vi "Startup 1.vi"(6 "LabVIEW Web Service":refnum<class "Web Service.lvclass">) -> ()   [LabVIEW 2015]
uses:
  <vilib>/wsapi/Web Service.lvclass
  Source/Classes/Request/Request.lvclass/Request.ctl
  Source/Classes/Request/Read method.vi
  Source/Classes/Request/Read params.vi
  <vilib>/National Instruments/JSON Support for LabVIEW/JSON Data Classes/JSON String/New JSON String.vi
  Source/Classes/Server/Add Response (Method Not Found from Request).vi
  Source/Classes/Server/Add Response (Result from Request).vi
  Source/Classes/Server/Add Response (Invalid Params from Request).vi
  <vilib>/National Instruments/JSON Support for LabVIEW/JSON Data Classes/JSON Datatype/To More Specific Type (Array).vi
  <vilib>/National Instruments/JSON Support for LabVIEW/JSON Data Classes/JSON Array/Index Array (Numeric).vi
  <vilib>/National Instruments/JSON Support for LabVIEW/JSON Data Classes/JSON Numeric/Read value (Numeric).vi
  <vilib>/National Instruments/JSON Support for LabVIEW/JSON Data Classes/JSON Numeric/New JSON Numeric.vi
  Source/Classes/Server/Add Response (Server Error from Request).vi
  <vilib>/National Instruments/JSON Support for LabVIEW/JSON Data Classes/JSON Datatype/JSON Datatype.lvclass
  Source/Classes/params/params.lvclass
  Source/Classes/Server/JSONRPC Server.lvclass
  Source/Classes/Request/Request.lvclass
  <vilib>/National Instruments/JSON Support for LabVIEW/JSON Data Classes/JSON Basic Type/JSON Basic Type.lvclass
  <vilib>/National Instruments/JSON Support for LabVIEW/JSON Data Classes/JSON Numeric/JSON Numeric.lvclass
  <vilib>/National Instruments/JSON Support for LabVIEW/JSON Data Classes/JSON String/JSON String.lvclass
  <vilib>/National Instruments/JSON Support for LabVIEW/JSON Data Classes/JSON Array/JSON Array.lvclass
panel:
  out "String":string
  in  "error in (no error)":errorcluster
  out "error out":errorcluster
  # "Use the web service input terminal to call the VIs on the Service subpalette of the Web Services palette. Do not remove it from the connector pane unless you don't need access to the palette."
  # "Any additional terminals added to the connector pane of a startup VI will be ignored."
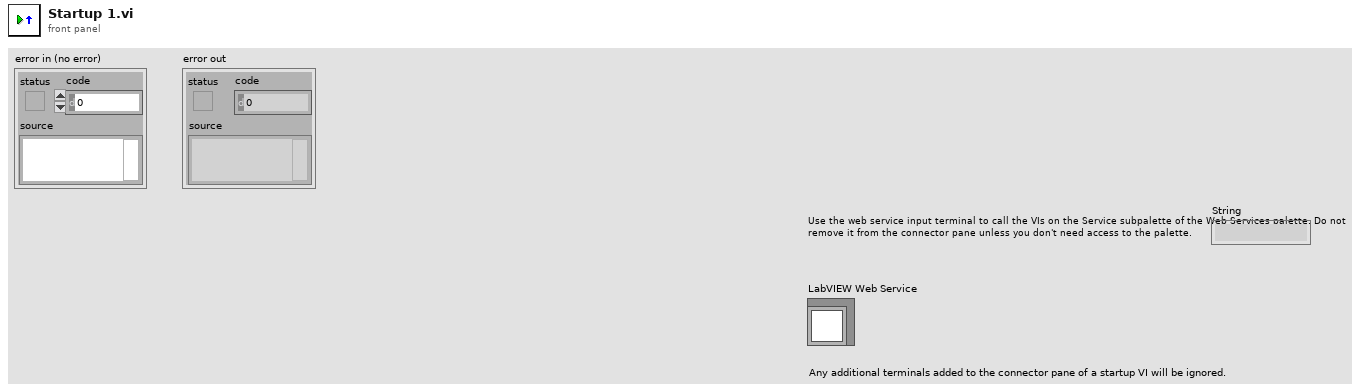
[diagram p1: front panel]
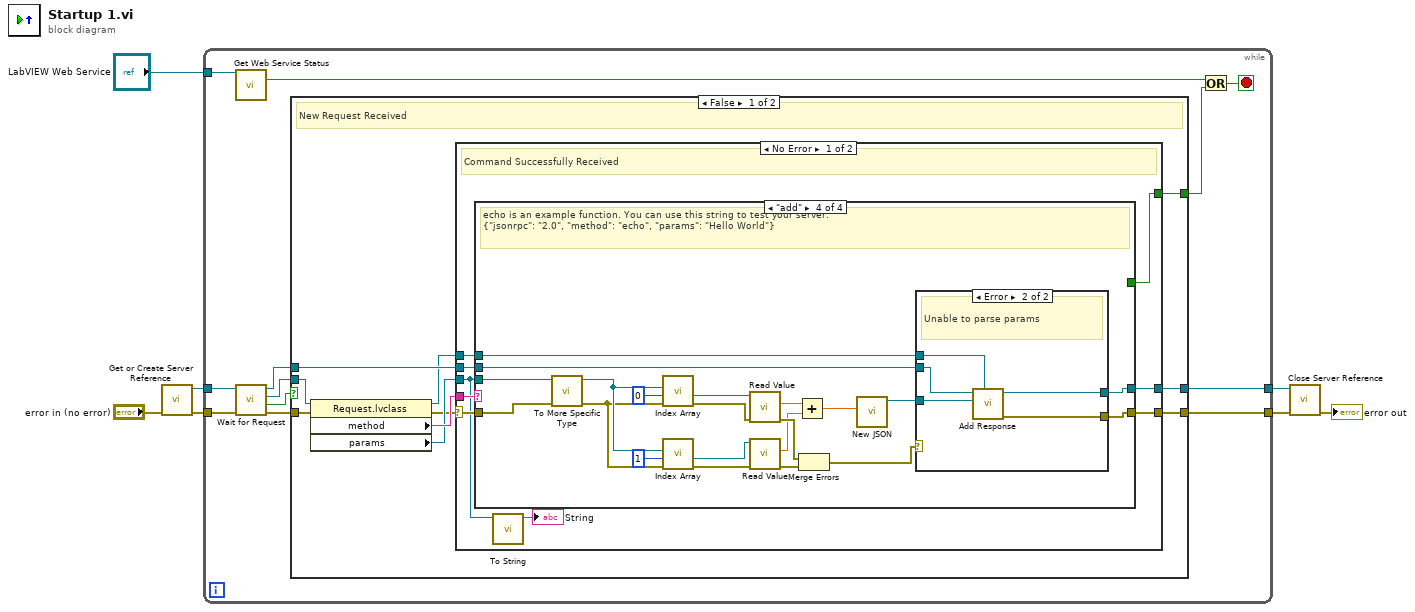
[diagram p0: block diagram]
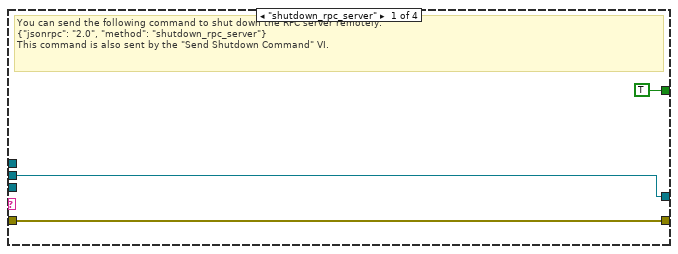
[diagram p2: hidden frame]
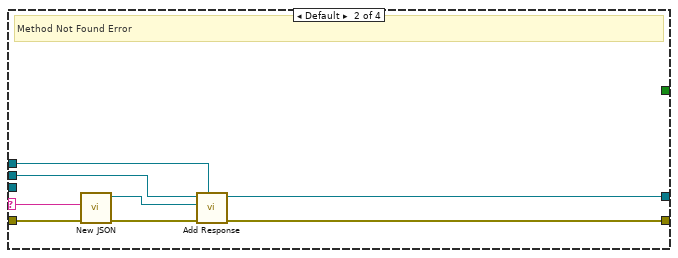
[diagram p3: hidden frame]
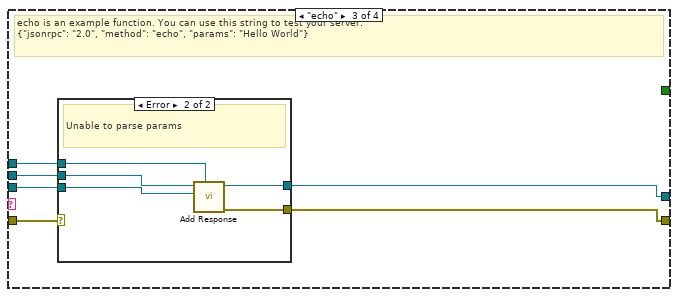
[diagram p4: hidden frame]
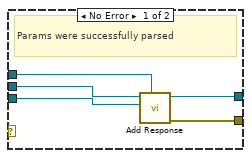
[diagram p5: hidden frame]
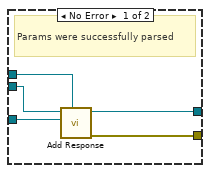
[diagram p6: hidden frame]
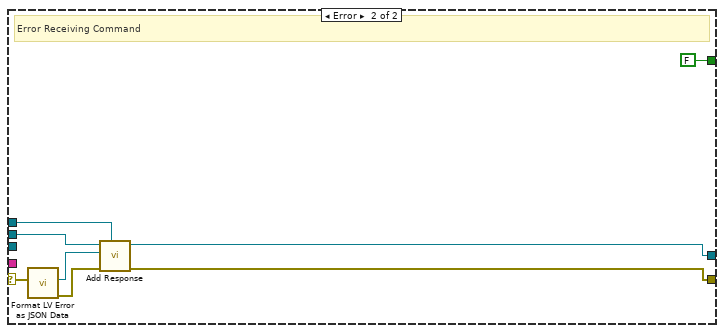
[diagram p7: hidden frame]
diagram:
  n1 = call "Get or Create Server Reference.vi"("error in (no error)"="error in (no error)") -> ("error out"=w6:errorcluster, "Server Out"=w7:refnum<class "JSONRPC Server.lvclass">)  [unwired: 9 in]
  n2 = while {
    tunnel: w7 -> [w19]
    tunnel: w6 -> [w15]
    tunnel: [w11] -> w4
    tunnel: [w13] -> w5
    tunnel: "LabVIEW Web Service" -> [w8]
    stop <- w10 stop-if-true
    n3 = call <vilib>:"Get Web Service Status.vi"("LabVIEW Web Service"=w8) -> ("service stopping?"=w9:bool)  [unwired: 12 in, 2 out]
    n4 = call "Wait for Request.vi"("error in (no error)"=w15, "Server in"=w19) -> ("error out"=w14:errorcluster, "timed out?"=w16:bool, "Request"=w17:refnum<class "Request.lvclass">, "Server out"=w18:refnum<class "JSONRPC Server.lvclass">)  [unwired: 6 in]
    n5 = case shown="False" w16 {
      tunnel: w18 -> [w22 w105]
      tunnel: w17 -> [w29 _]
      tunnel: w14 -> [w26 w106]
      tunnel: [w24 w106] -> w11
      tunnel: [w23 _] -> w12
      tunnel: [w21 w105] -> w13
      frame False {
        # "New Request Received"
        n6 = property class="Request.lvclass"(reference=w29, error in=w26) -> (reference out=w20:refnum<class "Request.lvclass">, error out=w25:errorcluster, "method"=w28:string, "params"=w27:refnum<class "JSON Datatype.lvclass">)
        n7 = case shown="No Error" w25 {
          selector: w25 -> [w37 w98]
          tunnel: w28 -> [w38 _]
          tunnel: w27 -> [w31 _]
          tunnel: [w36 w101] -> w24
          tunnel: [w35 FALSE] -> w23
          tunnel: w22 -> [w34 w103]
          tunnel: [w33 w102] -> w21
          tunnel: w20 -> [w32 w104]
          frame No Error {
            # "Command Successfully Received"
            n8 = case shown="\"add\"" w38 {
              selector: w38 -> [_ w45 _ _]
              tunnel: w31 -> [_ _ w51 w82]
              tunnel: w37 -> [w40 w44 w50 w80]
              tunnel: [w40 w47 w53 w84] -> w36
              tunnel: [TRUE _ _ _] -> w35
              tunnel: w34 -> [w39 w49 w55 w86]
              tunnel: [w39 w46 w54 w85] -> w33
              tunnel: w32 -> [_ w48 w52 w83]
              frame "shutdown_rpc_server" {
                # "You can send the following command to shut down the RPC server remotely:\n{\"jsonrpc\": \"2.0\", \"method\": \"shutdown_rpc_server\"}\nThis command is also sent by the \"Send Shutdown Command\" VI."
              }
              frame Default {
                # "Method Not Found Error"
                n9 = call-poly <vilib>:"New JSON.vi"("error in (no error)"=w44, "value"=w45) -> ("error out"=w43:errorcluster, "JSON String out"=w42:refnum<class "JSON String.lvclass">)  [unwired: 8 in]
                n10 = call-poly "Add Response.vi"("Request"=w48, "error in (no error)"=w43, "JSON in"=w42, "Server in"=w49) -> ("error out"=w47:errorcluster, "Server out"=w46:refnum<class "JSONRPC Server.lvclass">)  [unwired: 5 in, 1 out]
              }
              frame "echo" {
                # "echo is an example function. You can use this string to test your server:\n{\"jsonrpc\": \"2.0\", \"method\": \"echo\", \"params\": \"Hello World\"}"
                n11 = case shown="Error" w50 {
                  tunnel: w55 -> [w60 w65]
                  tunnel: [w59 w64] -> w54
                  tunnel: w51 -> [w58 w63]
                  tunnel: [w57 w62] -> w53
                  tunnel: w52 -> [w56 w61]
                  frame No Error {
                    # "Params were successfully parsed"
                    n12 = call-poly "Add Response.vi"("Request"=w56, "JSON in"=w58, "Server in"=w60) -> ("error out"=w57:errorcluster, "Server out"=w59:refnum<class "JSONRPC Server.lvclass">)  [unwired: 6 in, 1 out]
                  }
                  frame Error {
                    # "Unable to parse params"
                    n13 = call-poly "Add Response.vi"("Request"=w61, "JSON in"=w63, "Server in"=w65) -> ("error out"=w62:errorcluster, "Server out"=w64:refnum<class "JSONRPC Server.lvclass">)  [unwired: 6 in, 1 out]
                  }
                }
              }
              frame "add" {
                # "echo is an example function. You can use this string to test your server:\n{\"jsonrpc\": \"2.0\", \"method\": \"echo\", \"params\": \"Hello World\"}"
                n14 = call-poly <vilib>:"To More Specific Type.vi"("error in (no error)"=w80, "JSON Datatype in"=w82) -> ("error out"=w69:errorcluster, "JSON Datatype out"=w81:refnum<class "JSON Array.lvclass">)  [unwired: 8 in]
                n15 = call-poly <vilib>:"Index Array.vi"("error in (no error)"=w69, "index"=0, "JSON Array in"=w81) -> ("error out"=w68:errorcluster, "JSON Numeric"=w72:refnum<class "JSON Numeric.lvclass">)  [unwired: 7 in]
                n16 = call-poly <vilib>:"Index Array.vi"("error in (no error)"=w69, "index"=1, "JSON Array in"=w81) -> ("error out"=w70:errorcluster, "JSON Numeric"=w71:refnum<class "JSON Numeric.lvclass">)  [unwired: 7 in]
                n17 = call-poly <vilib>:"Read Value.vi"("error in (no error)"=w68, "JSON String in"=w72) -> ("error out"=w79:errorcluster, "value"=w76:dbl)  [unwired: 7 in, 1 out]
                n18 = call-poly <vilib>:"Read Value.vi"("error in (no error)"=w70, "JSON String in"=w71) -> ("error out"=w78:errorcluster, "value"=w75:dbl)  [unwired: 7 in, 1 out]
                n19 = Add(x=w76, y=w75) -> (x+y=w74:dbl)
                n20 = Merge Errors(w79, w78) -> (w77:errorcluster)
                n21 = call-poly <vilib>:"New JSON.vi"("value"=w74) -> ("JSON String out"=w73:refnum<class "JSON Numeric.lvclass">)  [unwired: 9 in, 1 out]
                n22 = case shown="Error" w77 {
                  tunnel: w86 -> [w91 w96]
                  tunnel: [w90 w95] -> w85
                  tunnel: w73 -> [w89 w94]
                  tunnel: [w88 w93] -> w84
                  tunnel: w83 -> [w87 w92]
                  frame No Error {
                    # "Params were successfully parsed"
                    n23 = call-poly "Add Response.vi"("Request"=w87, "JSON in"=w89, "Server in"=w91) -> ("error out"=w88:errorcluster, "Server out"=w90:refnum<class "JSONRPC Server.lvclass">)  [unwired: 6 in, 1 out]
                  }
                  frame Error {
                    # "Unable to parse params"
                    n24 = call-poly "Add Response.vi"("Request"=w92, "JSON in"=w94, "Server in"=w96) -> ("error out"=w93:errorcluster, "Server out"=w95:refnum<class "JSONRPC Server.lvclass">)  [unwired: 6 in, 1 out]
                  }
                }
              }
            }
            n25 = call-dynamic "To String.vi"("JSON Datatype in"=w31) -> ("String"=→"String":string)  [unwired: 9 in, 1 out]
          }
          frame Error {
            # "Error Receiving Command"
            n26 = call "Format LV Error as JSON Data.vi"("error in"=w98) -> ("error out"=w99:errorcluster, "Error Object Out"=w97:refnum<class "JSON Object.lvclass">)  [unwired: 9 in]
            n27 = call-poly "Add Response.vi"("Request"=w104, "error in (no error)"=w99, "JSON in"=w97, "Server in"=w103) -> ("error out"=w101:errorcluster, "Server out"=w102:refnum<class "JSONRPC Server.lvclass">)  [unwired: 5 in, 1 out]
          }
        }
      }
      frame True {
        # "Timeout while waiting for new Requests"
      }
    }
    n28 = Or(x=w9, y=w12) -> (x .or. y?=w10:bool)
  }
  n29 = call-dynamic "Close Server Reference.vi"("error in (no error)"=w4, "Server in"=w5) -> ("error out"=→"error out":errorcluster)  [unwired: 9 in]
